vi "Test Example API.vi"() -> ()   [LabVIEW 2018]
doc: "Example API Tester."
uses:
  Example.lvlib
panel:
  in  "Get Bitness Info":bool
  in  "Append Trace":bool=TRUE
  in  "wait for reply":bool=TRUE
  in  "Show Block Diagram":bool
  in  "X":dbl=1.0
  out "Reply Payload":dbl
  in  "Stop Module":bool
  in  "Start Module":bool
  out "Do Something Count":i32
  in  "Test Do Something Else and Wait for Reply":bool
  in  "Hide Module Panel":bool
  in  "Show Module Panel":bool
  in  "Test Do Something Else":bool
  in  "Test Do Something":bool
  out "Status":string
  out "Module Running?":bool
  # "This VI tests the API for the Module."
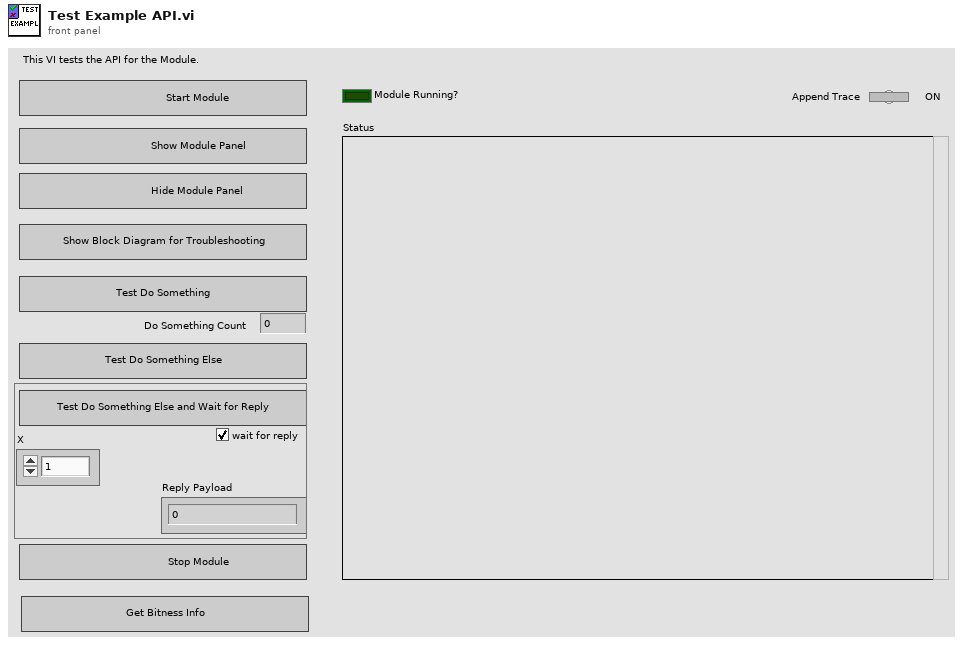
[diagram p1: front panel]
types:
  T1 = typedef "Example.lvlib/Broadcast Events--cluster.ctl" = cluster{"Module Did Init":refnum<user-event>, "Status Updated":refnum<user-event>, "Error Reported":refnum<user-event>, "Did Something":refnum<user-event>, "Module Did Stop":refnum<user-event>, "Update Module Execution Status":refnum<user-event>}
  T2 = typedef "Example.lvlib/Do Something Else and Wait (Reply Payload)--cluster.ctl" = cluster{"Value":dbl, "error":errorcluster}
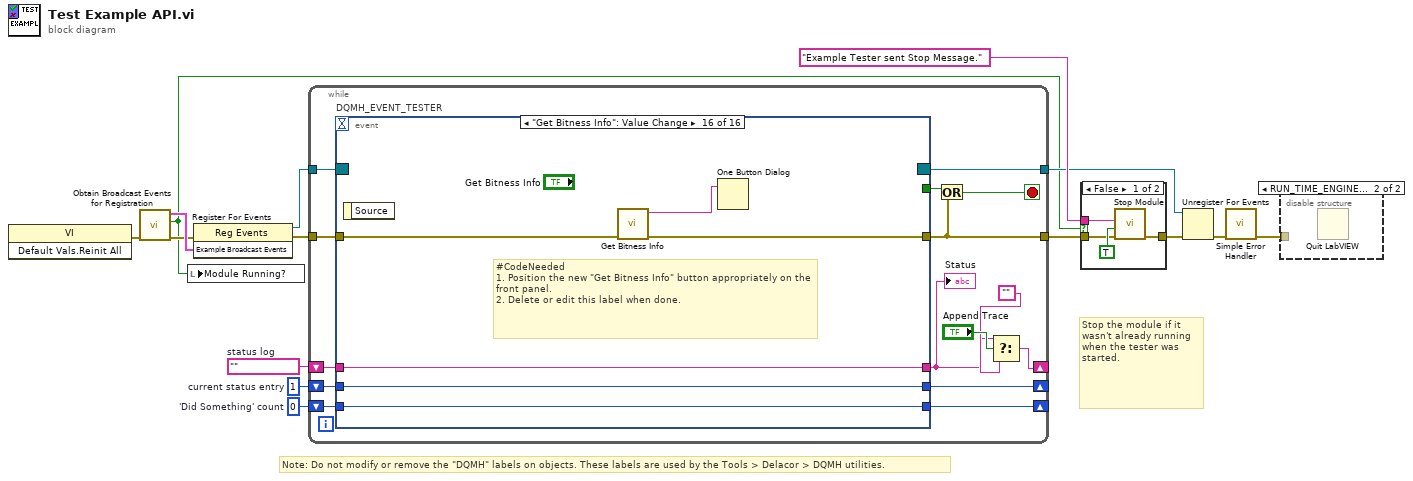
[diagram p0: block diagram]
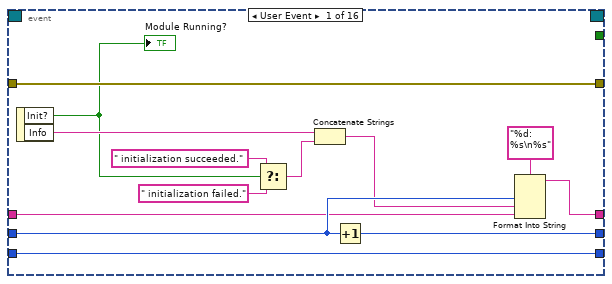
[diagram p3: hidden frame]
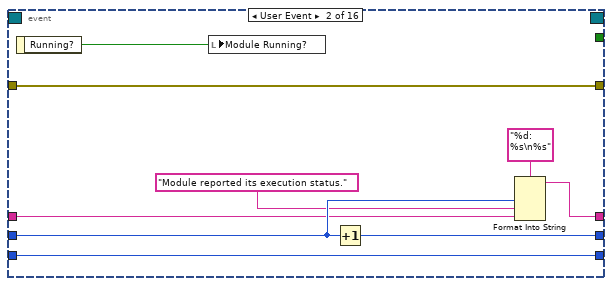
[diagram p4: hidden frame]
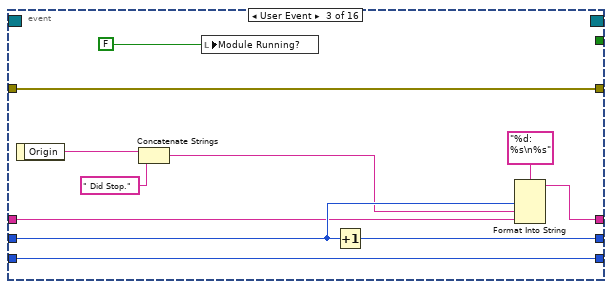
[diagram p5: hidden frame]
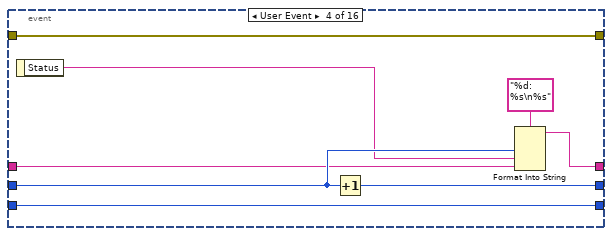
[diagram p6: hidden frame]
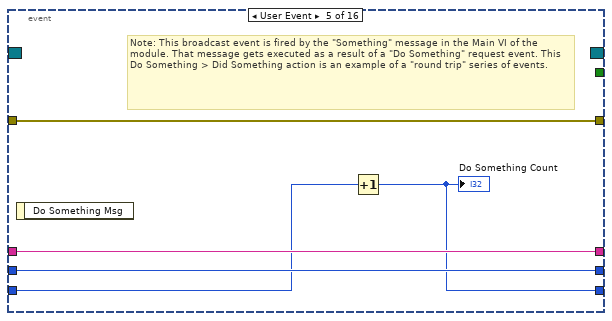
[diagram p7: hidden frame]
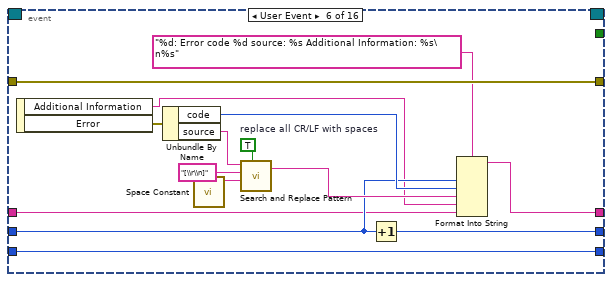
[diagram p8: hidden frame]
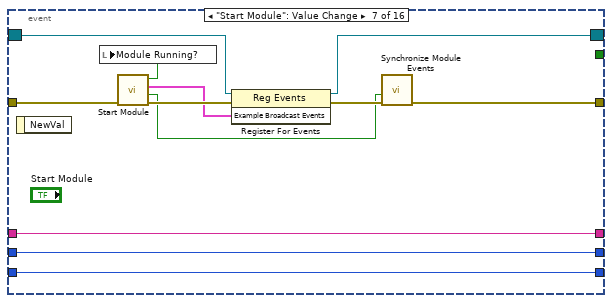
[diagram p9: hidden frame]
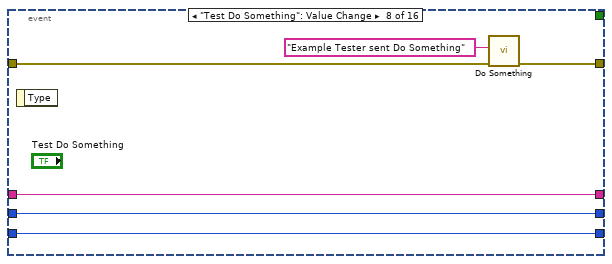
[diagram p10: hidden frame]
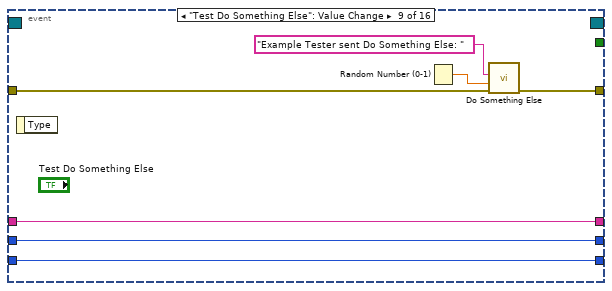
[diagram p11: hidden frame]
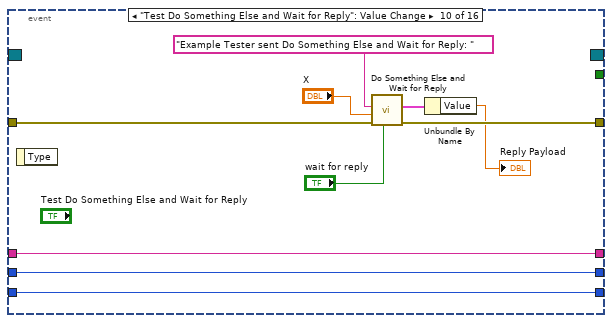
[diagram p12: hidden frame]
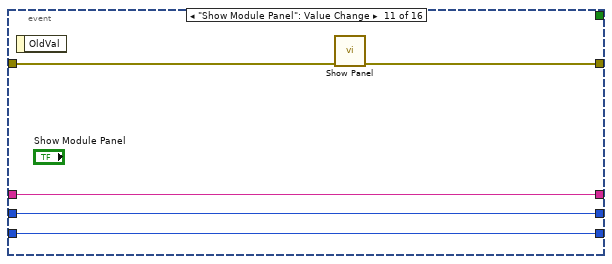
[diagram p13: hidden frame]
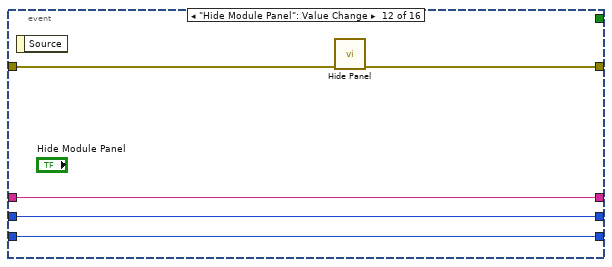
[diagram p14: hidden frame]
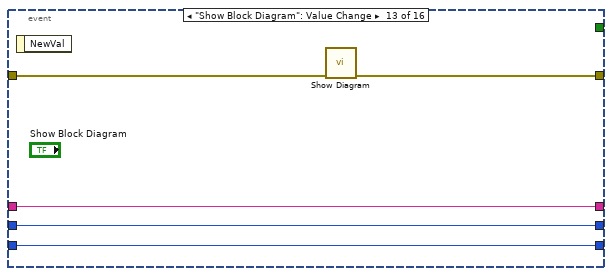
[diagram p15: hidden frame]
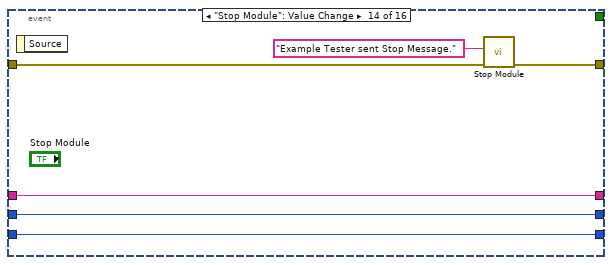
[diagram p16: hidden frame]
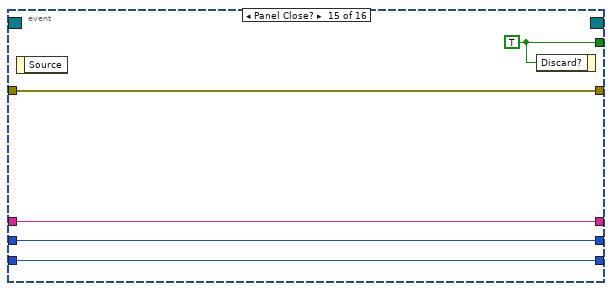
[diagram p17: hidden frame]
diagram:
  w11 = 0  # 'Did Something' count
  w12 = 1  # current status entry
  w13 = ""  # status log
  # "Stop the module if it wasn't already running when the tester was started."
  # "Note: Do not modify or remove the \"DQMH\" labels on objects. These labels are used by the Tools > Delacor > DQMH utilities."
  n1 = invoke class="VI" method="Default Vals.Reinit All"() -> (error out=w6:errorcluster)  [unwired: 3 in, 2 out]
  n2 = call "Obtain Broadcast Events for Registration.vi"("error in (no error)"=w6) -> ("error out"=w5:errorcluster, "Already running?"=w4:bool, "Example Broadcast Events"=w9:T1)  [unwired: 8 in]
  n3 = local write "Module Running?"(w4) -> ()
  n4 = register-events(error in=w5, w9) -> (reference out=w8:refnum<event-registration>, error out=w10:errorcluster)  [unwired: 1 in]
  n5 = while {
    tunnel: w8 -> [w30]
    tunnel: [w20] -> w3
    shift-right: [w18] -> _
    shift-left: w13 -> [w27]
    shift-right: [w26] -> _
    shift-left: w12 -> [w28]
    shift-right: [w24] -> _
    shift-left: w11 -> [w25]
    tunnel: w10 -> [w22]
    tunnel: [w21] -> w7
    stop <- w23 stop-if-true
    n6 = event "DQMH_EVENT_TESTER" shown="[15] \"Get Bitness Info\": Value Change" {
      selector: w30 -> [_ _ _ _ _ _ w96 _ _ _ _ _ _ _ _ _]
      dyn-events: [_ _ _ _ _ _ w95 _ _ _ _ _ _ _ _ _] -> w21
      timeout: _ -> [_ _ _ _ _ _ _ _ _ _ _ _ _ _ _ _]
      tunnel: [_ _ _ _ _ _ _ _ _ _ _ _ _ _ w152 _] -> w29
      tunnel: [w43 w46 w54 w65 w72 w90 w94 w109 w116 w126 w131 w136 w137 w144 w148 w154] -> w20
      tunnel: w28 -> [w41 w51 w62 w68 w75 w80 w100 w106 w112 w123 w129 w134 w139 w146 w150 w156]
      tunnel: w27 -> [w31 w44 w53 w64 w76 w77 w101 w107 w113 w124 w130 w135 w140 w147 w151 w157]
      tunnel: [w39 w49 w60 w69 w76 w81 w101 w107 w113 w124 w130 w135 w140 w147 w151 w157] -> w16
      tunnel: [w40 w50 w61 w71 w75 w79 w100 w106 w112 w123 w129 w134 w139 w146 w150 w156] -> w26
      tunnel: w25 -> [w36 w47 w56 w66 w74 w91 w99 w105 w111 w122 w128 w133 w138 w145 w149 w155]
      tunnel: [w36 w47 w56 w66 w73 w91 w99 w105 w111 w122 w128 w133 w138 w145 w149 w155] -> w24
      tunnel: w22 -> [w43 w46 w54 w65 w72 w90 w93 w104 w110 w119 w127 w132 w141 w142 w148 w158]
      event User Event {
        n7 = event-data() -> ("Init?"=w35:bool, "Info"=w38:string)  [unwired: 1 in]
        "Module Running?" <- w35
        n8 = Select(t=" initialization succeeded.", s=w35, f=" initialization failed.") -> (s? t:f=w32:string)
        n9 = Concatenate Strings(w38, w32) -> (w37:string)
        n10 = Increment(x=w41) -> (x+1=w40:i32)
        n11 = Format Into String(format string="%d: %s\n%s", w41, w37, w31) -> (resulting string=w39:string)  [unwired: 2 in, 1 out]
      }
      event User Event {
        n12 = event-data() -> ("Running?"=w45:bool)  [unwired: 1 in]
        n13 = local write "Module Running?"(w45) -> ()
        n14 = Increment(x=w51) -> (x+1=w50:i32)
        n15 = Format Into String(format string="%d: %s\n%s", w51, "Module reported its execution status.", w44) -> (resulting string=w49:string)  [unwired: 2 in, 1 out]
      }
      event User Event {
        n16 = event-data() -> ("Origin"=w59:string)  [unwired: 1 in]
        n17 = Concatenate Strings(w59, " Did Stop.") -> (w58:string)
        n18 = local write "Module Running?"(FALSE ("Module Did Init?")) -> ()
        n19 = Increment(x=w62) -> (x+1=w61:i32)
        n20 = Format Into String(format string="%d: %s\n%s", w62, w58, w53) -> (resulting string=w60:string)  [unwired: 2 in, 1 out]
      }
      event User Event {
        n21 = event-data() -> ("Status"=w67:string)  [unwired: 1 in]
        n22 = Increment(x=w68) -> (x+1=w71:i32)
        n23 = Format Into String(format string="%d: %s\n%s", w68, w67, w64) -> (resulting string=w69:string)  [unwired: 2 in, 1 out]
      }
      event User Event {
        # "Note: This broadcast event is fired by the \"Something\" message in the Main VI of the module. That message gets executed as a result of a \"Do Something\" request event. This Do Something > Did Something action is an example of a \"round trip\" series of events."
        n24 = event-data() -> ()  [unwired: 1 in, 1 out]
        n25 = Increment(x=w74) -> (x+1=w73:i32)
        "Do Something Count" <- w73
      }
      event User Event {
        w86 = TRUE  # replace all CR/LF with spaces
        n26 = event-data() -> ("Additional Information"=w78:string, "Error"=w82:errorcluster)  [unwired: 1 in]
        n27 = Unbundle By Name(w82) -> ("code"=w83:i32, "source"=w84:string)
        n28 = call <vilib>:"Space Constant.vi"() -> ("String"=w87:string)
        n29 = call <vilib>:"Search and Replace Pattern.vi"("string"=w84, "regular expression (\"\")"="[\\r\\n]" ("regular expression (\"\")"), "replace string (\"\")"=w87, "replace all? (F)"=w86) -> ("result string"=w85:string)  [unwired: 1 in, 1 out]
        n30 = Increment(x=w80) -> (x+1=w79:i32)
        n31 = Format Into String(format string="%d: Error code %d source: %s Additional Information: %s\n%s", w80, w83, w85, w78, w77) -> (resulting string=w81:string)  [unwired: 2 in, 1 out]
      }
      event "Start Module": Value Change {
        n32 = event-data() -> ()  [unwired: 1 in, 1 out]
        n33 = call "Start Module.vi"("error in (no error)"=w93) -> ("error out"=w102:errorcluster, "Wait for Event Sync?"=w98:bool, "Example Broadcast Events"=w97:T1, "Module Was Already Running?"=w92:bool)  [unwired: 7 in]
        n34 = local write "Module Running?"(w92) -> ()
        n35 = register-events(reference=w96, error in=w102, w97) -> (reference out=w95:refnum<event-registration>, error out=w103:errorcluster)
        n36 = call "Synchronize Module Events.vi"("error in"=w103, "Wait for Event Sync?"=w98) -> ("error out"=w94:errorcluster)  [unwired: 9 in]
      }
      event "Test Do Something": Value Change {
        n37 = event-data() -> ()  [unwired: 1 in, 1 out]
        n38 = call "Do Something.vi"("error in (no error)"=w104, "Do Something Message"="Example Tester sent Do Something") -> ("error out"=w109:errorcluster)  [unwired: 9 in]
      }
      event "Test Do Something Else": Value Change {
        n39 = event-data() -> ()  [unwired: 1 in, 1 out]
        n40 = Random Number (0-1)() -> (number: 0 to 1=w114:dbl)
        n41 = call "Do Something Else.vi"("error in (no error)"=w110, "X"=w114, "Do Something Else Message"="Example Tester sent Do Something Else: " ("Do Something Message")) -> ("error out"=w116:errorcluster)  [unwired: 8 in]
      }
      event "Test Do Something Else and Wait for Reply": Value Change {
        n42 = event-data() -> ()  [unwired: 1 in, 1 out]
        n43 = call "Do Something Else and Wait for Reply.vi"("wait for reply (T)"="wait for reply", "error in (no error)"=w119, "X"="X", "Do Something Else Message"="Example Tester sent Do Something Else and Wait for Reply: " ("Do Something Message")) -> ("error out"=w126:errorcluster, "Reply Payload"=w121:T2)  [unwired: 5 in, 1 out]
        n44 = Unbundle By Name(w121) -> ("Value"=→"Reply Payload":dbl)
      }
      event "Show Module Panel": Value Change {
        n45 = event-data() -> ()  [unwired: 1 in, 1 out]
        n46 = call "Show Panel.vi"("error in (no error)"=w127) -> ("error out"=w131:errorcluster)  [unwired: 10 in]
      }
      event "Hide Module Panel": Value Change {
        n47 = event-data() -> ()  [unwired: 1 in, 1 out]
        n48 = call "Hide Panel.vi"("error in (no error)"=w132) -> ("error out"=w136:errorcluster)  [unwired: 10 in]
      }
      event "Show Block Diagram": Value Change {
        n49 = event-data() -> ()  [unwired: 1 in, 1 out]
        n50 = call "Show Diagram.vi"("error in (no error)"=w141) -> ("error out"=w137:errorcluster)  [unwired: 10 in]
      }
      event "Stop Module": Value Change {
        n51 = event-data() -> ()  [unwired: 1 in, 1 out]
        n52 = call "Stop Module.vi"("error in"=w142, "Origin"="Example Tester sent Stop Message.") -> ("error out"=w144:errorcluster)  [unwired: 9 in]
      }
      event Panel Close? {
        w152 = TRUE ("Discard?")
        n53 = event-data() -> ()  [unwired: 1 in, 1 out]
        n54 = event-data("Discard?"=w152) -> ()  [unwired: 1 in, 1 out]
      }
      event "Get Bitness Info": Value Change {
        # "#CodeNeeded\n1. Position the new \"Get Bitness Info\" button appropriately on the front panel.\n2. Delete or edit this label when done."
        n55 = event-data() -> ()  [unwired: 1 in, 1 out]
        n56 = call "Get Bitness Info.vi"("error in"=w158) -> ("error out"=w154:errorcluster, "BitnessInfo"=w153:string)  [unwired: 8 in, 1 out]
        n57 = One Button Dialog(message=w153) -> ()  [unwired: 1 in, 1 out]
      }
    }
    "Status" <- w16
    n58 = Or(x=w29, y=w20) -> (x .or. y?=w23:bool)
    n59 = Select(t=w16, s="Append Trace", f="") -> (s? t:f=w18:string)
  }
  n60 = case shown="False" w4 {
    tunnel: [w162 w163] -> w15
    tunnel: "Example Tester sent Stop Message." ("Origin") -> [w161 _]
    tunnel: w3 -> [w159 w163]
    frame False {
      n61 = call "Stop Module.vi"("error in"=w159, "Wait for Module to Stop? (F)"=TRUE ("Wait for Module to stop?"), "Origin"=w161) -> ("error out"=w162:errorcluster)  [unwired: 8 in]
    }
    frame True {
    }
  }
  n62 = Unregister For Events(event registration refnum=w7, error in=w15) -> (error out=w2:errorcluster)
  n63 = call <vilib>:"Simple Error Handler.vi"("error in (no error)"=w2) -> ("error out"=w1:errorcluster)  [unwired: 4 in, 4 out]
  n64 = disable-structure shown="RUN_TIME_ENGINE==True" {
    disable-tunnel: w1 -> [_ _]
    frame condition #0 (active) {
    }
    frame condition #1 {
      n65 = Quit LabVIEW() -> ()  [unwired: 1 in]
    }
  }
